vi "usrp_stream_tx.vi"() -> ()   [LabVIEW 2014]
uses:
  <vilib>/addons/Modulation/Digital/General/MT Generate Bits (Galois, PN Order).vi
  <vilib>/addons/Modulation/Analog/support/mod_Set Error Source.vi
  <vilib>/addons/Modulation/Digital/Support/Common/Validators/mod_Generate Bits Validate.vi
  var_stop.vi
  <vilib>/addons/Modulation/Digital/Support/Common/Validators/mod_Generate Filter Coefficients Validate.vi
  <vilib>/addons/Modulation/Digital/General/subVIs/mod_Generate Filter Coefficients.vi
  <vilib>/addons/Modulation/Digital/General/MT Generate PSK System Parameters(M).vi
  <vilib>/addons/Modulation/Digital/General/subVIs/mod_Generate Bits PN Sequence.vi
  <vilib>/addons/Modulation/Digital/General/MT Map Bits to PSK Symbols.vi
  <vilib>/addons/Modulation/Digital/General/MT Apply Pulse Shaping Filter (Generic).vi
  <instrlib>/niUSRP/niUSRP Write Tx Data (CDB Cluster).vi
  <vilib>/addons/Modulation/niDMT.lvlib
panel:
  out "error out":errorcluster
  in  "pulse shaping samples per symbol (16)":i32=4 caption="pulse shaping samples per symbol"
  in  "stop":bool
  in  "Enabled Channels":string(combo)="0"
  in  "Timebase Clock Source":string(combo)="Internal"
  in  "Frequency Source":string(combo)="Internal"
  out "coerced gain":dbl format="%#_6f"
  out "coerced carrier frequency":dbl=100000.0 format="%#_6p"
  out "coerced IQ rate":dbl=100000.0 format="%#_6p"
  in  "active antenna":string="TX1"
  in  "gain":dbl=10.0 format="%#_6f"
  in  "carrier frequency":dbl=915000000.0 format="%#_6p"
  in  "device names":refnum<k15>="192.168.10.3"
  in  "IQ rate":dbl=1000000.0 format="%#_6p"
  # "This is an point-to-point communication link prototype\nfor streaming mode USRPs\n\nThis program is developed by Teng-Hui Huang, Network Information and Communications Laboratory, NTU Taiwan.\n\nQuick Start:\n1. Connect USRPs to PCs\n2. Run usrp_stream_rx.vi\n3. Run usrp_stream_tx.vi\n\nIf there is any issues, please send an e-mail to me\nhui811116@outlook.com\nTeng-Hui Huang. Nov. 19. 2017."
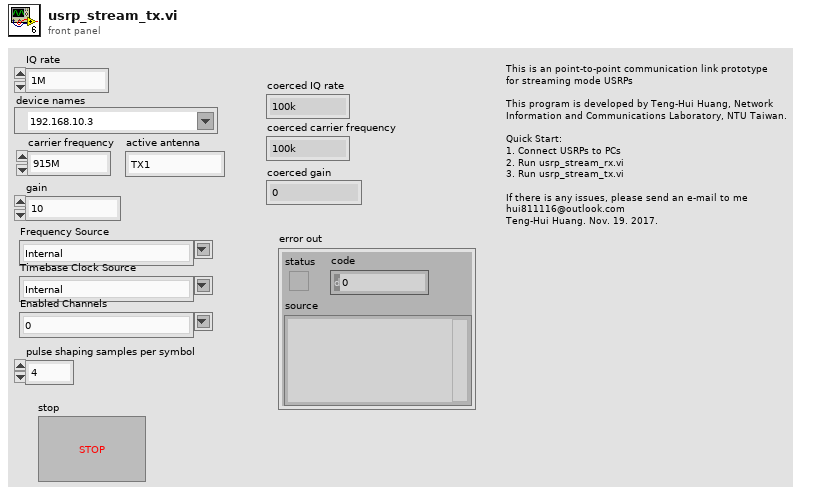
[diagram p1: front panel]
types:
  T1 = enum16{"none", "Raised Cosine", "Root Raised Cos", "Gaussian"}
  T2 = enum16{"FSK", "PSK", "QAM", "MSK", "PAM", "ASK", "CPM"}
  T3 = cluster{"samples per symbol (16)":i32, "symbol map":cdb[], "differential PSK":enum16{"disable", "enable"}, "PSK type":u16}
  T4 = typedef "niAMT.lvlib/Complex Data Waveform.ctl" = cluster{"t0":dbl, "dt":dbl, "Y":cdb[]}
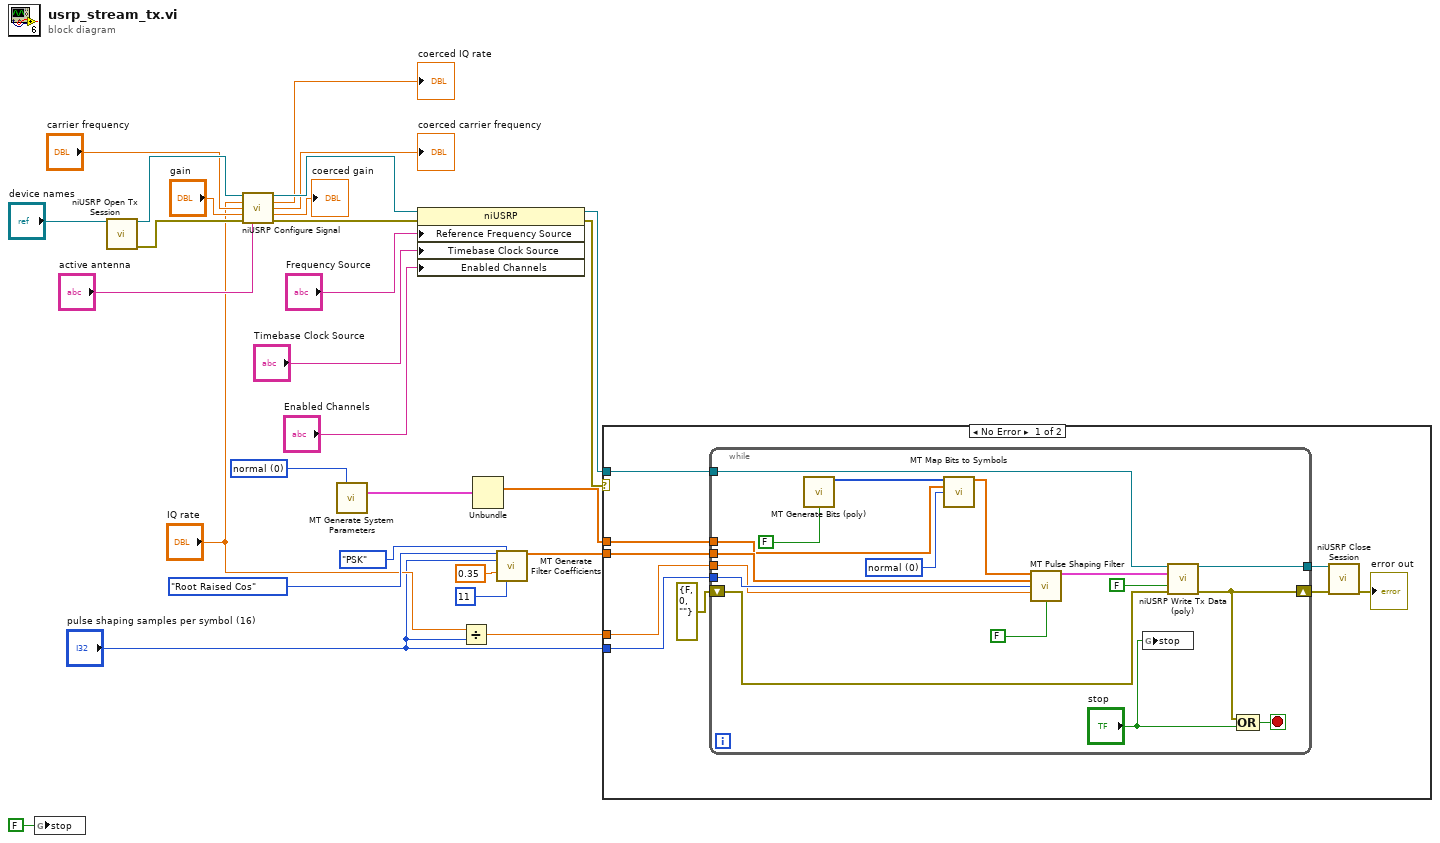
[diagram p0: block diagram]
diagram:
  w3 = u16 0 items=["normal", "shifted", "offset"] ("PSK type")
  n1 = global write "var_stop.vi" "stop"(FALSE) -> ()
  n2 = call <instrlib>:"niUSRP Open Tx Session.vi"("device names"="device names") -> ("session handle out"=w28:refnum<k15>, "error out"=w27:errorcluster)  [unwired: 13 in]
  n3 = call <instrlib>:"niUSRP Configure Signal.vi"("session handle"=w28, "IQ rate"="IQ rate", "carrier frequency"="carrier frequency", "gain"="gain", "error in (no error)"=w27, "active antenna"="active antenna") -> ("session handle out"=w22:refnum<k15>, "coerced IQ rate"=→"coerced IQ rate":dbl, "coerced carrier frequency"=→"coerced carrier frequency":dbl, "coerced gain"=→"coerced gain":dbl, "error out"=w21:errorcluster)  [unwired: 5 in]
  n4 = call-poly <vilib>:"MT Generate System Parameters.vi"("PSK type"=w3) -> ("PSK system parameters"=w2:T3)  [unwired: 12 in, 2 out]
  n5 = property class="niUSRP"(reference=w22, error in=w21, "Reference Frequency Source"="Frequency Source", "Timebase Clock Source"="Timebase Clock Source", "Enabled Channels"="Enabled Channels") -> (reference out=w14:refnum<k15>, error out=w4:errorcluster)
  n6 = Divide(x="IQ rate", y="pulse shaping samples per symbol (16)") -> (x/y=w5:dbl)
  n7 = Unbundle(w2) -> ("symbol map"=w1:cdb[])  [unwired: 3 out]
  n8 = call <vilib>:"MT Generate Filter Coefficients.vi"("pulse shaping filter (none)"=T1."Root Raised Cos", "modulation type"=T2."PSK", "pulse shaping samples per symbol (16)"="pulse shaping samples per symbol (16)", "filter parameter"=0.35, "filter length (symbols)"=11) -> ("pulse shaping filter coefficients"=w8:dbl[])  [unwired: 8 in, 2 out]
  n9 = case shown="No Error" w4 {
    tunnel: w14 -> [w37 _]
    tunnel: w8 -> [w31 _]
    tunnel: "pulse shaping samples per symbol (16)" -> [w33 _]
    tunnel: w5 -> [w32 _]
    tunnel: w1 -> [w29 _]
    frame No Error {
      n10 = while {
        tunnel: w37 -> [w54]
        tunnel: [w53] -> w36
        shift-right: [w47] -> w35
        shift-left: errorcluster {"status"=FALSE, "code"=0, "source"=""} ("error out") -> [w52]
        tunnel: w33 -> [w46]
        tunnel: w32 -> [w45]
        tunnel: w31 -> [w43]
        tunnel: w29 -> [w39]
        stop <- w51 stop-if-true
        w40 = u16 0 items=["normal", "shifted", "offset"] ("PSK type")
        n11 = call-poly <vilib>:"MT Generate Bits (poly).vi"("reset? (T)"=FALSE) -> ("output bit stream"=w41:i8[])  [unwired: 12 in, 2 out]
        n12 = call-poly <vilib>:"MT Map Bits to Symbols.vi"("input bit stream"=w41, "symbol map"=w39, "PSK type"=w40) -> ("symbols"=w38:cdb[])  [unwired: 11 in, 1 out]
        n13 = call-poly <vilib>:"MT Pulse Shaping Filter.vi"("symbols"=w38, "pulse shaping filter coefficients"=w43, "samples per symbol (16)"=w46, "symbol rate (Hz)"=w45, "reset? (T)"=FALSE) -> ("output complex waveform"=w48:T4)  [unwired: 9 in, 1 out]
        n14 = global write "var_stop.vi" "stop"("stop") -> ()
        n15 = call-poly <instrlib>:"niUSRP Write Tx Data (poly).vi"("session handle"=w54, "data"=w48, "end of data?"=FALSE, "error in (no error)"=w52) -> ("session handle out"=w53:refnum<k15>, "error out"=w47:errorcluster)  [unwired: 10 in]
        n16 = Compound Arithmetic op=OR(w47, "stop") -> (w51:bool)
      }
      n17 = call <instrlib>:"niUSRP Close Session.vi"("session handle"=w36, "error in (no error)"=w35) -> ("error out"=→"error out":errorcluster)  [unwired: 13 in]
    }
    frame Error {
    }
  }
